vi "Actor Core.vi"(8 "error in":errorcluster, 11 "UIActor in":refnum<class "MusicManagerActor.lvclass">) -> (0 "error out":errorcluster, 3 "Actor out":refnum<class "Actor.lvclass">)   [LabVIEW 2015, in "MusicManagerActor.lvlib" / "MusicManagerActor.lvclass"]
doc: "(<B>Filename</B>: Actor Framework.lvlib:Actor.lvclass:Actor Core.vi)\n\nReceives messages to the actor, reacts to them, and initiates any error handling that may shut the actor down.\n\nDescendant classes may override this VI to append parallel tasks for the actor to complete while it handles messages. Overrides use the Call Parent Method node."
uses:
  MusicManagerActor.lvclass
  <vilib>/ActorFramework/Actor/Actor.lvclass
  MusicManagerActor.lvclass/MusicManagerActor.ctl
  <vilib>/ActorFramework/Message Enqueuer/Message Enqueuer.lvclass/Message Enqueuer.ctl
  <vilib>/ActorFramework/Message Enqueuer/Enqueue.vi
  <vilib>/ActorFramework/Message Priority Queue/Priority Enqueue.vi
  <vilib>/ActorFramework/Stop Msg/Stop Msg.lvclass
  MusicManagerActor Messages/View Album Library Request Msg/View Album Library Request Msg.lvclass
  MusicManagerActor Messages/View Artist Library Request Msg/View Artist Library Request Msg.lvclass
  MusicManagerActor Messages/View Song Library Request Msg/View Song Library Request Msg.lvclass
  MusicManagerActor Messages/View Song Queue Request Msg/View Song Queue Request Msg.lvclass
  MusicManagerActor Messages/Search Song Library Msg/Search Song Library Msg.lvclass
panel:
  in  "Main UI":enum32{"Main", "Debug"}(tab)
  in  "Search String":string
  in  "Queue":bool
  in  "Albums":bool
  in  "Artists":bool
  in  "Songs":bool
  # "Your Music"
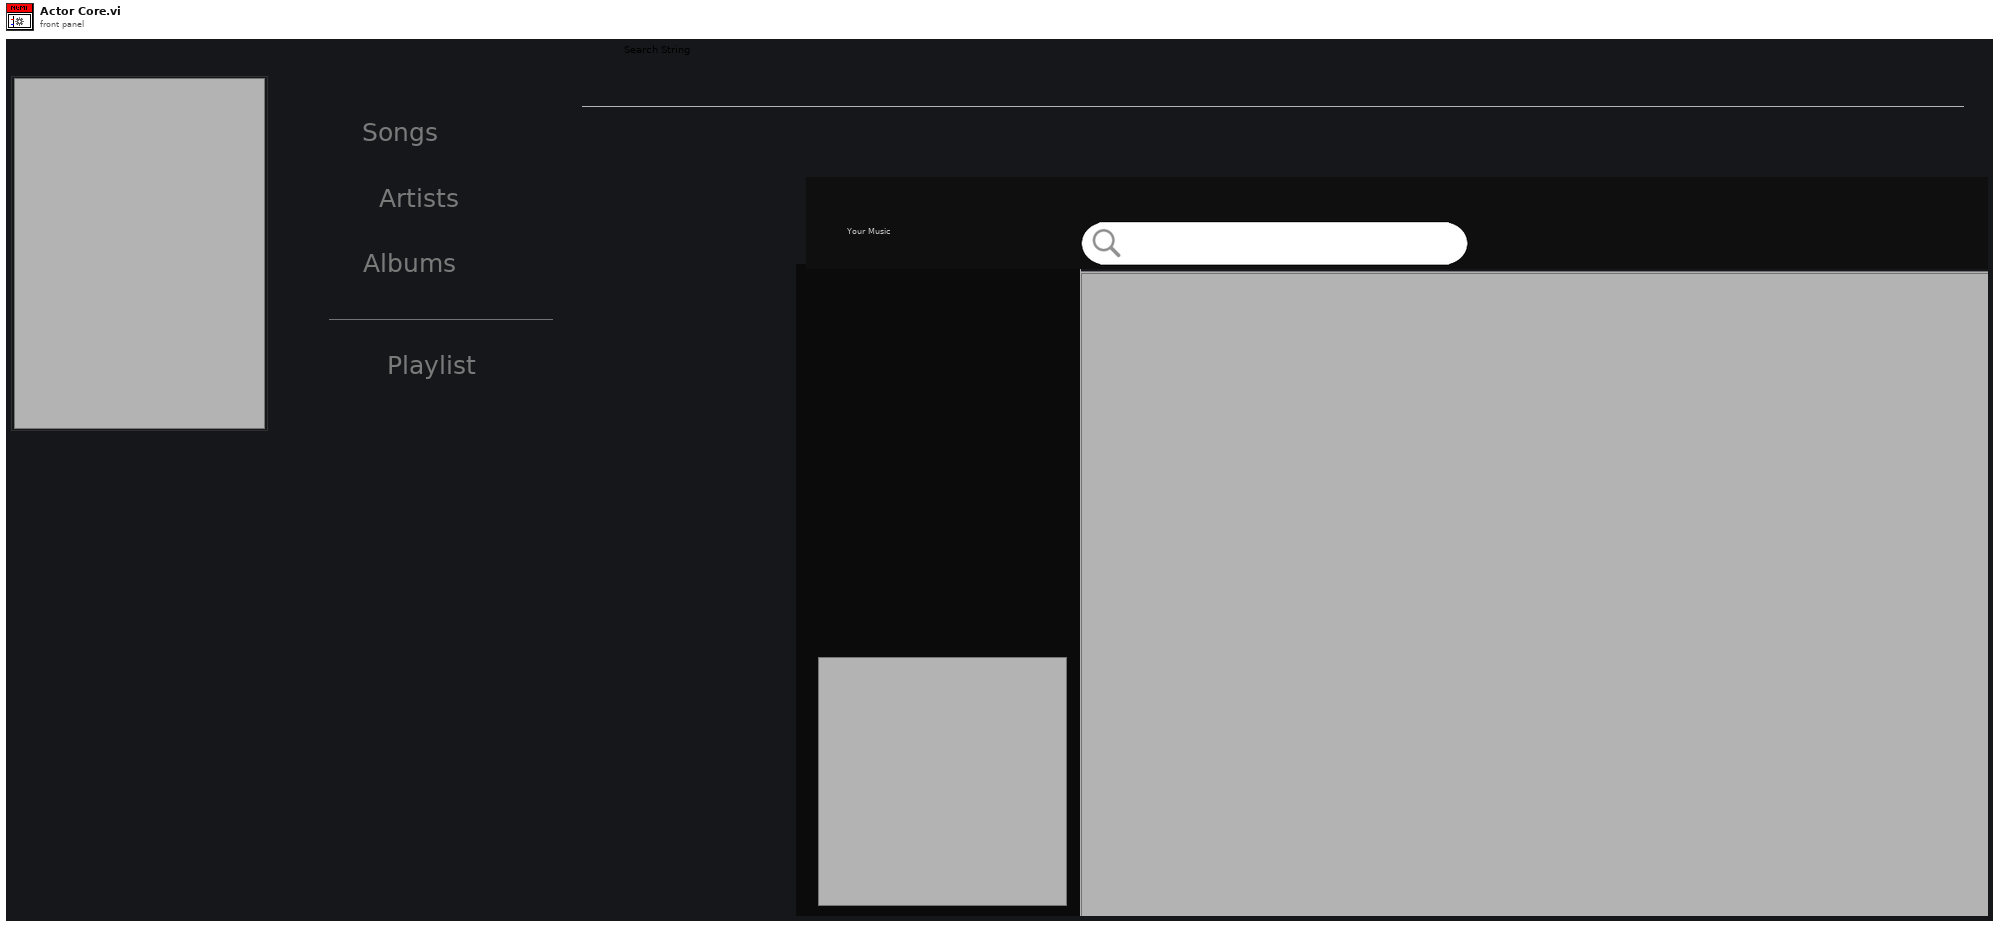
[diagram p1: front panel]
types:
  T1 = typedef "MusicManagerActor.lvlib/MusicManagerActor.lvclass/Nested Actors Enqueuers.ctl" = cluster{"Self Enqueuer":refnum<class "Message Enqueuer.lvclass">, "Song Queue":refnum<class "Message Enqueuer.lvclass">, "Song Browser":refnum<class "Message Enqueuer.lvclass">, "Album Image Manager":refnum<class "Message Enqueuer.lvclass">}
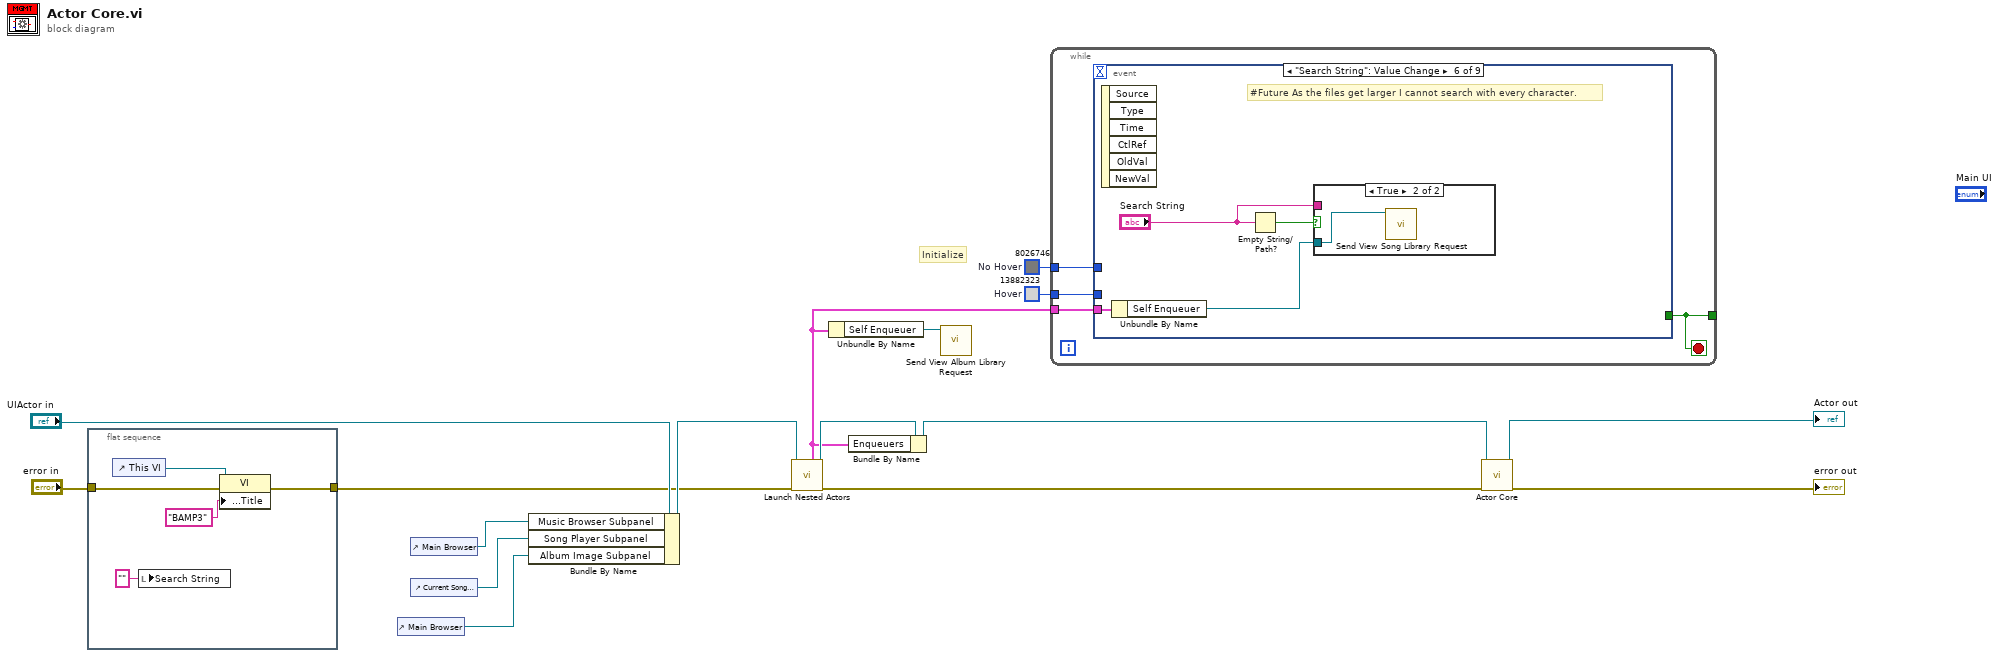
[diagram p0: block diagram]
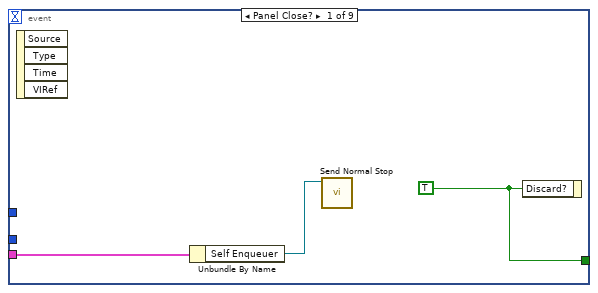
[diagram p2: hidden frame]
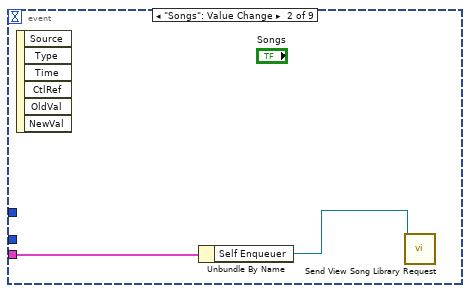
[diagram p3: hidden frame]
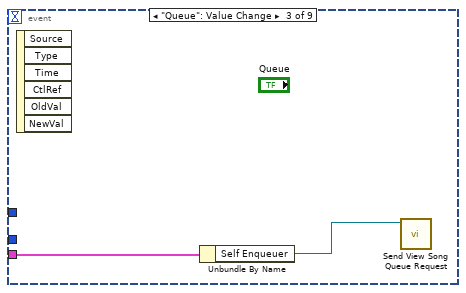
[diagram p4: hidden frame]
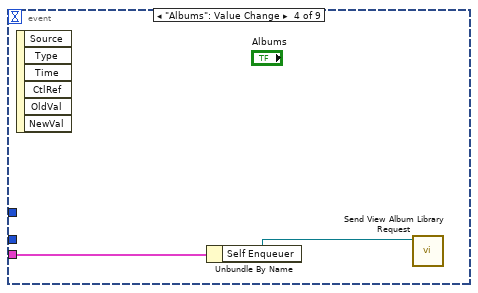
[diagram p5: hidden frame]
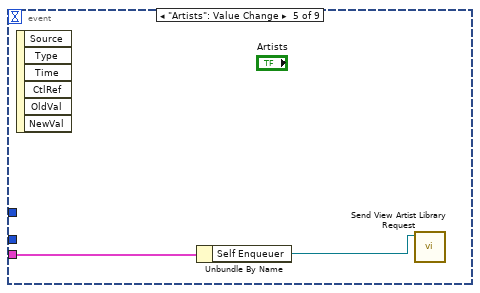
[diagram p6: hidden frame]
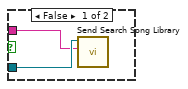
[diagram p7: hidden frame]
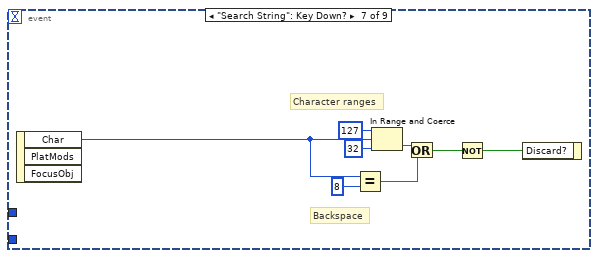
[diagram p8: hidden frame]
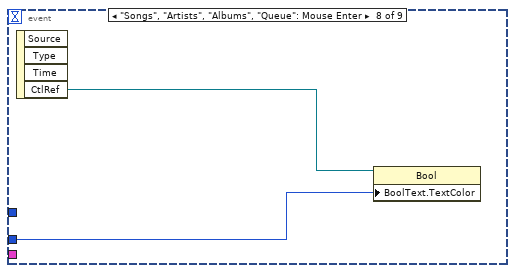
[diagram p9: hidden frame]
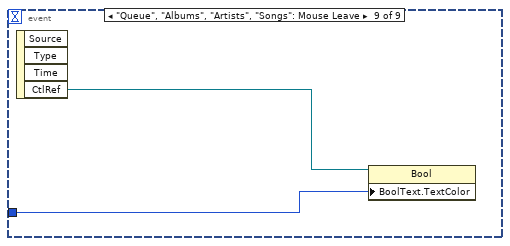
[diagram p10: hidden frame]
diagram:
  w11 = u32 13882323  # Hover
  w10 = u32 8026746  # No Hover
  # "Initialize"
  n1 = flat-sequence {
    tunnel: "error in" -> [w20]
    tunnel: [w19] -> w4
    frame #0 {
      n2 = control-ref of="This VI"() -> (w18:refnum<vi>)
      n3 = local write "Search String"("" ("Search String")) -> ()
      n4 = property class="VI"(reference=w18, error in=w20, "Front Panel.Title"="BAMP3" ("Front Panel Window:Title")) -> (error out=w19:errorcluster)  [unwired: 1 out]
    }
  }
  n5 = control-ref of="Main Browser"() -> (w1:refnum<vi>)
  n6 = control-ref of="Main Browser"() -> (w8:refnum<vi>)
  n7 = control-ref of="Current Song Subpanel"() -> (w7:refnum<vi>)
  n8 = Bundle By Name(cluster="UIActor in", "Music Browser Subpanel"=w8, "Song Player Subpanel"=w7, "Album Image Subpanel"=w1) -> (w9:refnum<class "MusicManagerActor.lvclass">)
  n9 = call "Launch Nested Actors.vi"("error in (no error)"=w4, "MusicManagerActor in"=w9) -> ("error out"=w3:errorcluster, "MusicManagerActor out"=w14:refnum<class "MusicManagerActor.lvclass">, "Nested Actor Enqueuers"=w2:T1)  [unwired: 7 in]
  n10 = Unbundle By Name(w2) -> ("Self Enqueuer"=w12:refnum<class "Message Enqueuer.lvclass">)
  n11 = Bundle By Name(cluster=w14, "Enqueuers"=w2) -> (w13:refnum<class "MusicManagerActor.lvclass">)
  n12 = call "Send View Album Library Request.vi"("Message Enqueuer in"=w12) -> ()  [unwired: 9 in, 2 out]
  n13 = while {
    tunnel: w2 -> [w25]
    tunnel: w11 -> [w24]
    tunnel: w10 -> [w23]
    tunnel: [w22] -> _
    stop <- w22 stop-if-true
    n14 = event shown="[5] \"Search String\": Value Change" {
      selector: _ -> [_ _ _ _ _ _ _ _ _]
      dyn-events: _ -> [_ _ _ _ _ _ _ _ _]
      timeout: _ -> [_ _ _ _ _ _ _ _ _]
      tunnel: [w28 _ _ _ _ _ _ _ _] -> w22
      tunnel: w25 -> [w27 w30 w32 w34 w36 w39 _ _ _]
      tunnel: w24 -> [_ _ _ _ _ _ _ w52 _]
      tunnel: w23 -> [_ _ _ _ _ _ _ _ w54]
      event Panel Close? {
        w28 = TRUE ("Discard?")
        n15 = event-data() -> ()  [unwired: 1 in, 4 out]
        n16 = Unbundle By Name(w27) -> ("Self Enqueuer"=w26:refnum<class "Message Enqueuer.lvclass">)
        n17 = call <vilib>:"Send Normal Stop.vi"("Message Enqueuer"=w26) -> ()  [unwired: 10 in, 1 out]
        n18 = event-data("Discard?"=w28) -> ()  [unwired: 1 in, 1 out]
      }
      event "Songs": Value Change {
        n19 = event-data() -> ()  [unwired: 1 in, 6 out]
        n20 = Unbundle By Name(w30) -> ("Self Enqueuer"=w29:refnum<class "Message Enqueuer.lvclass">)
        n21 = call "Send View Song Library Request.vi"("Message Enqueuer in"=w29) -> ()  [unwired: 9 in, 2 out]
      }
      event "Queue": Value Change {
        n22 = event-data() -> ()  [unwired: 1 in, 6 out]
        n23 = Unbundle By Name(w32) -> ("Self Enqueuer"=w31:refnum<class "Message Enqueuer.lvclass">)
        n24 = call "Send View Song Queue Request.vi"("Message Enqueuer in"=w31) -> ()  [unwired: 9 in, 2 out]
      }
      event "Albums": Value Change {
        n25 = event-data() -> ()  [unwired: 1 in, 6 out]
        n26 = Unbundle By Name(w34) -> ("Self Enqueuer"=w33:refnum<class "Message Enqueuer.lvclass">)
        n27 = call "Send View Album Library Request.vi"("Message Enqueuer in"=w33) -> ()  [unwired: 9 in, 2 out]
      }
      event "Artists": Value Change {
        n28 = event-data() -> ()  [unwired: 1 in, 6 out]
        n29 = Unbundle By Name(w36) -> ("Self Enqueuer"=w35:refnum<class "Message Enqueuer.lvclass">)
        n30 = call "Send View Artist Library Request.vi"("Message Enqueuer in"=w35) -> ()  [unwired: 9 in, 2 out]
      }
      event "Search String": Value Change {
        # "#Future As the files get larger I cannot search with every character."
        n31 = event-data() -> ()  [unwired: 1 in, 6 out]
        n32 = Unbundle By Name(w39) -> ("Self Enqueuer"=w38:refnum<class "Message Enqueuer.lvclass">)
        n33 = Empty String/Path?(string/path="Search String") -> (empty?=w40:bool)
        n34 = case shown="True" w40 {
          tunnel: w38 -> [w42 w43]
          tunnel: "Search String" -> [w41 _]
          frame False {
            n35 = call "Send Search Song Library.vi"("Search String"=w41, "Message Enqueuer in"=w42) -> ()  [unwired: 8 in, 2 out]
          }
          frame True {
            n36 = call "Send View Song Library Request.vi"("Message Enqueuer in"=w43) -> ()  [unwired: 9 in, 2 out]
          }
        }
      }
      event "Search String": Key Down? {
        # "Backspace"
        # "Character ranges"
        n37 = event-data() -> ("Char"=w49:i16)  [unwired: 1 in, 2 out]
        n38 = Equal?(x=w49, y=i16 8) -> (x = y?=w47:bool)
        n39 = In Range and Coerce(upper limit=i16 127, x=w49, lower limit=i16 32) -> (In Range?=w46:bool)  [unwired: 1 out]
        n40 = Or(x=w46, y=w47) -> (x .or. y?=w45:bool)
        n41 = Not(x=w45) -> (.not. x?=w44:bool)
        n42 = event-data("Discard?"=w44) -> ()  [unwired: 1 in, 1 out]
      }
      event "Songs", "Artists", "Albums", "Queue": Mouse Enter {
        n43 = event-data() -> ("CtlRef"=w53:refnum<vi>)  [unwired: 1 in, 3 out]
        n44 = property class="Bool"(reference=w53, "BoolText.TextColor"=w52) -> ()  [unwired: 1 in, 2 out]
      }
      event "Queue", "Albums", "Artists", "Songs": Mouse Leave {
        n45 = event-data() -> ("CtlRef"=w55:refnum<vi>)  [unwired: 1 in, 3 out]
        n46 = property class="Bool"(reference=w55, "BoolText.TextColor"=w54) -> ()  [unwired: 1 in, 2 out]
      }
    }
  }
  n47 = call-parent "Actor Core.vi"("error in"=w3, "Actor in"=w13) -> ("error out"=→"error out":errorcluster, "Actor out"=→"Actor out":refnum<class "Actor.lvclass">)  [unwired: 8 in]
